vi "WSVCAP SHL FPGA LL Procedure RFFE - Bus Park.vi"(0 "Procedure Step":T1, 1 "Wait Ticks Remaining":u32, 5 "Wait Ticks":u32, 11 "error in (no error)":errorcluster, 13 "Socket Mask":u32) -> (3 "Wait Ticks Remaining Out":u32, 4 "Procedure Step Out":T1, 10 "Finished":bool, 15 "error out":errorcluster)   [LabVIEW 2012]
uses:
  Type Defs/WSVCAP SHL Procedure Step Enum.ctl
  Type Defs/WSVCAP SHL RFFE Write Line Enum.ctl
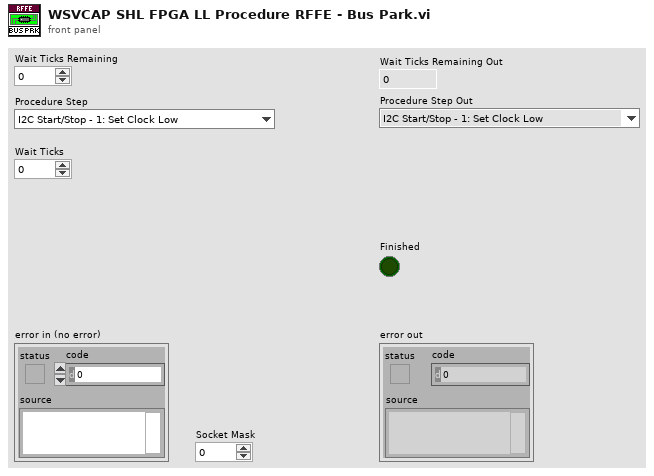
[diagram p1: front panel]
types:
  T1 = typedef "WSVCAP SHL Procedure Step Enum.ctl" = enum16{"I2C Start/Stop - 1: Set Clock Low", "I2C Start/Stop - 2: Wait", "I2C Start/Stop - 3: Set Data I", "I2C Start/Stop - 4: Wait", "I2C Start/Stop - 5: Set Clock High", "I2C Start/Stop - 6: Wait", "I2C Start/Stop - 7: Set Data II", "I2C Start/Stop - 8: Wait", "I2C Start/Stop - 9: Set Clock Low", "I2C Start/Stop - 10: Wait", "I2C Read ACK - 1: Set Clock High", "I2C Read ACK - 2: Wait", "I2C Read ACK - 3: Read ACK Bit", "I2C Read ACK - 4: Wait", "I2C Read ACK - 5: Set Clock Low", "I2C Read ACK - 6: Wait", "I2C Write ACK - 1: Write ACK Bit", "I2C Write ACK - 2: Wait", "I2C Write ACK - 3: Set Clock High", "I2C Write ACK - 4: Wait", "I2C Write ACK - 5: Set Clock Low", "I2C Write ACK - 6: Wait", "I2C Write ACK - 7: Set Data Low", "I2C Send Add - 1: Reset Bits Remaining", "I2C Send Add - 2: Set Data Bit", "I2C Send Add - 3: Wait", "I2C Send Add - 4: Set Clock High", "I2C Send Add - 5: Wait", "I2C Send Add - 6: Set Clock Low", "I2C Send Add - 7: Wait", "I2C Send Add - 8: Check Bits Remaining", "I2C Send Data - 1: Reset Bits Remaining", "I2C Send Data - 2: Load Write Bit from FIFO", "I2C Send Data - 3: Set Data Bit", "I2C Send Data - 4: Wait", "I2C Send Data - 5: Set Clock High", "I2C Send Data - 6: Wait", "I2C Send Data - 7: Set Clock Low", "I2C Send Data - 8: Wait", "I2C Send Data - 9: Check Bits Remaining", "I2C Receive Data - 1: Reset Bits Remaining", "I2C Receive Data - 2: Wait", "I2C Receive Data - 3: Set Clock High", "I2C Receive Data - 4: Wait", "I2C Receive Data - 5: Read Data Bit", "I2C Receive Data - 6: Wait", "I2C Receive Data - 7: Set Clock Low", "I2C Receive Data - 8: Wait", "I2C Receive Data - 9: Check Bits Remaining", "SPI Clear Lines - 1:Clear", "SPI Send/Receive - 1: Load SDA - Clock Low", "SPI Send/Receive - 2: Wait", "SPI Send/Receive - 3: Load DATO - Clock High", "SPI Send/Receive - 4: Wait", "SPI Wait CMD Delay - 1:Wait", "RFFE Send SSC - 1:Set Low", "RFFE Send SSC - 2:Wait", "RFFE Send SSC - 3:Set SDA High", "RFFE Send SSC - 4:Wait", "RFFE Send SSC - 5:Set SDA Low", "RFFE Send SSC - 6:Wait", "RFFE Send Data - 1:Set SCL High", "RFFE Send Data - 2:Wait", "RFFE Send Data - 3:Set SCL Low", "RFFE Send Data - 4:Wait", "RFFE Send Data - 5:Set SCL High (P)", "RFFE Send Data - 6:Wait", "RFFE Send Data - 7:Set SCL Low (P)", "RFFE Send Data - 8:Wait", "RFFE Send Data - 9:Set SCL High (BP)", "RFFE Send Data - 10:Wait", "RFFE Send Data - 11:Set SCL Low (BP)", "RFFE Send Data - 12:Wait", "RFFE Receive Data - 1:Set SCL High", "RFFE Receive Data - 2:Wait", "RFFE Receive Data - 3:Set SCL Low", "RFFE Receive Data - 4:Wait", "RFFE Receive Data - 5:Set SCL High (BP)", "RFFE Receive Data - 6:Wait", "RFFE Receive Data - 7:Set SCL Low (BP)", "RFFE Receive Data - 8:Wait", "RFFE Bus Park - 1:Set SCL High", "RFFE Bus Park - 2:Wait", "RFFE Bus Park - 3:Set SCL Low", "RFFE Bus Park - 4:Wait", "RFFE Wait CMD Delay - 1:Wait", "RFFE Clear Lines - 1:Clear"}
  T2 = typedef "WSVCAP SHL RFFE Write Line Enum.ctl" = enum16{"SDAA", "SCLK"}
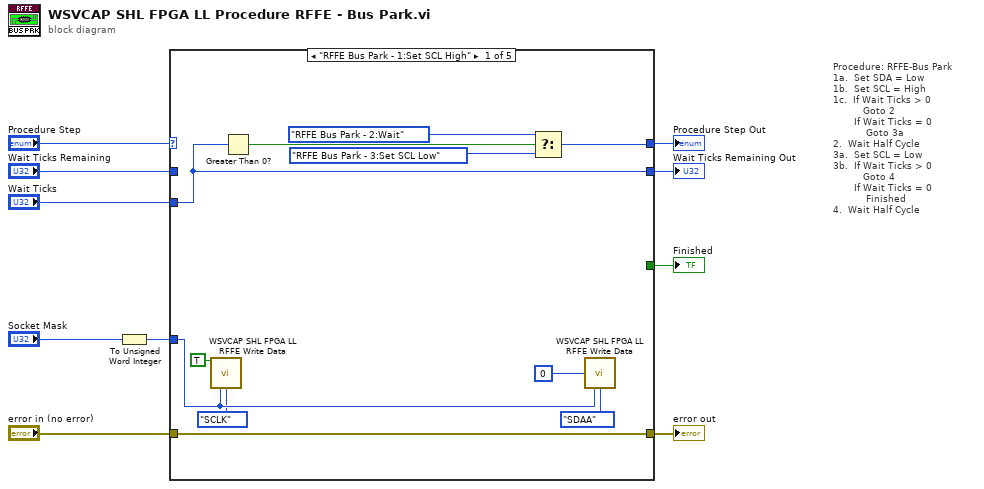
[diagram p0: block diagram]
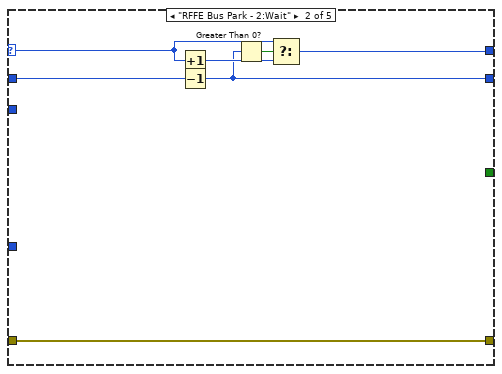
[diagram p2: hidden frame]
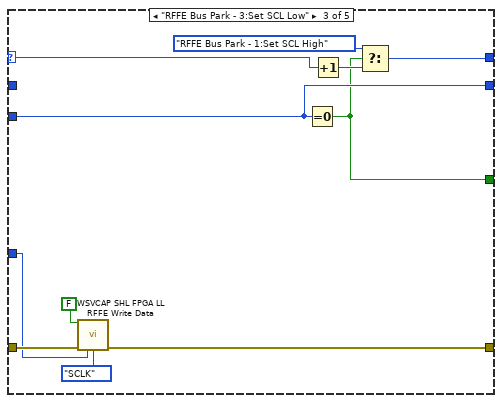
[diagram p3: hidden frame]
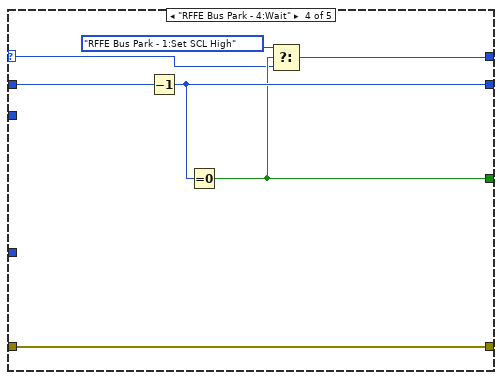
[diagram p4: hidden frame]
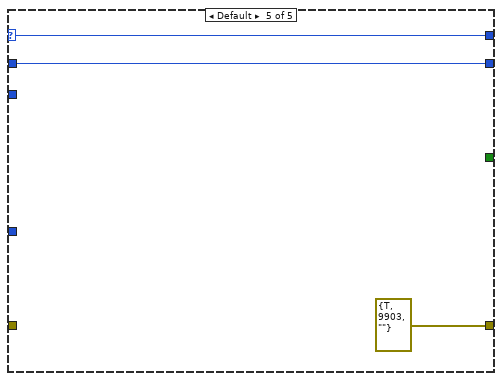
[diagram p5: hidden frame]
diagram:
  # "Procedure: RFFE-Bus Park\n1a.  Set SDA = Low\n1b.  Set SCL = High\n1c.  If Wait Ticks > 0\n          Goto 2\n       If Wait Ticks = 0 \n           Goto 3a\n2.  Wait Half Cycle\n3a.  Set SCL = Low\n3b.  If Wait Ticks > 0\n          Goto 4\n       If Wait Ticks = 0 \n           Finished\n4.  Wait Half Cycle"
  n1 = To Unsigned Word Integer(number="Socket Mask") -> (unsigned 16bit integer=w7:u16)
  n2 = case shown="\"RFFE Bus Park - 1:Set SCL High\"" "Procedure Step" {
    selector: "Procedure Step" -> [_ w26 w39 w40 w48]
    tunnel: [w19 w28 w35 w46 errorcluster {"status"=TRUE, "code"=9903, "source"=""} ("error IO")] -> w9
    tunnel: "error in (no error)" -> [w19 w28 w36 w46 _]
    tunnel: "Wait Ticks Remaining" -> [_ w24 _ w45 w47]
    tunnel: "Wait Ticks" -> [w15 _ w31 _ _]
    tunnel: [_ _ w29 w42 _] -> w8
    tunnel: w7 -> [w14 _ w34 _ _]
    tunnel: [w16 w23 w32 w44 w48] -> w2
    tunnel: [w15 w22 w31 w43 w47] -> w1
    frame "RFFE Bus Park - 1:Set SCL High" {
      n3 = call "WSVCAP SHL FPGA LL RFFE Write Data.vi"("CLK In"=TRUE ("Bit In"), "Socket Mask"=w14, "Line"=WSVCAP_SHL_RFFE_Write_Line_Enum."SCLK") -> ()  [unwired: 12 in, 1 out]
      n4 = Greater Than 0?(x=w15) -> (x > 0?=w20:bool)
      n5 = Select(t=WSVCAP_SHL_Procedure_Step_Enum."RFFE Bus Park - 2:Wait" ("Procedure Step"), s=w20, f=WSVCAP_SHL_Procedure_Step_Enum."RFFE Bus Park - 3:Set SCL Low" ("Procedure Step")) -> (s? t:f=w16:T1)
      n6 = call "WSVCAP SHL FPGA LL RFFE Write Data.vi"("Data Word In"=u16 0 ("Data Out"), "Socket Mask"=w14, "Line"=WSVCAP_SHL_RFFE_Write_Line_Enum."SDAA") -> ()  [unwired: 12 in, 1 out]
    }
    frame "RFFE Bus Park - 2:Wait" {
      n7 = Increment(x=w26) -> (x+1=w25:T1)
      n8 = Decrement(x=w24) -> (x-1=w22:u32)
      n9 = Greater Than 0?(x=w22) -> (x > 0?=w27:bool)
      n10 = Select(t=w26, s=w27, f=w25) -> (s? t:f=w23:T1)
    }
    frame "RFFE Bus Park - 3:Set SCL Low" {
      n11 = call "WSVCAP SHL FPGA LL RFFE Write Data.vi"("CLK In"=FALSE ("Bit In"), "error in (no error)"=w36, "Socket Mask"=w34, "Line"=WSVCAP_SHL_RFFE_Write_Line_Enum."SCLK") -> ("error out"=w35:errorcluster)  [unwired: 11 in]
      n12 = Equal To 0?(x=w31) -> (x = 0?=w29:bool)
      n13 = Increment(x=w39) -> (x+1=w38:T1)
      n14 = Select(t=WSVCAP_SHL_Procedure_Step_Enum."RFFE Bus Park - 1:Set SCL High" ("Procedure Step"), s=w29, f=w38) -> (s? t:f=w32:T1)
    }
    frame "RFFE Bus Park - 4:Wait" {
      n15 = Decrement(x=w45) -> (x-1=w43:u32)
      n16 = Equal To 0?(x=w43) -> (x = 0?=w42:bool)
      n17 = Select(t=WSVCAP_SHL_Procedure_Step_Enum."RFFE Bus Park - 1:Set SCL High" ("f"), s=w42, f=w40) -> (s? t:f=w44:T1)
    }
    frame Default {
    }
  }
  "error out" <- w9
  "Finished" <- w8
  "Procedure Step Out" <- w2
  "Wait Ticks Remaining Out" <- w1
